vi "MFC Parse.vi"(1 "MFC Raw":fxp<+/-,24,9>[](array[numeric])=[0.0, 0.0, 0.0, 0.0, 0.0, 0.0, 0.0, 0.0, 0.0, 0.0, 0.0, 0.0, 0.0, 0.0, 0.0, 0.0, 0.0, 0.0, 0.0, 0.0, 0.0, 0.0, 0.0, 0.0, 0.0, 0.0, 0.0, 0.0, 0.0, 0.0, 0.0, 0.0, 0.0, 0.0, 0.0, 0.0, 0.0, 0.0, 0.0, 0.0, 0.0, 0.0, 0.0, 0.0, 0.0, 0.0, 0.0, 0.0, 0.0, 0.0, 0.0, 0.0, 0.0, 0.0, 0.0, 0.0, 0.0, 0.0, 0.0, 0.0, 0.0, 0.0, 0.0, 0.0, 0.0, 0.0, 0.0, 0.0, 0.0, 0.0, 0.0, 0.0, 0.0, 0.0, 0.0, 0.0, 0.0, 0.0, 0.0, 0.0, 0.0, 0.0, 0.0, 0.0, 0.0, 0.0, 0.0, 0.0, 0.0, 0.0, 0.0, 0.0, 0.0, 0.0, 0.0, 0.0, 0.0, 0.0, 0.0, 0.0, 0.0, 0.0, 0.0, 0.0, 0.0, 0.0, 0.0, 0.0, 0.0, 0.0, 0.0, 0.0, 0.0, 0.0, 0.0, 0.0, 0.0, 0.0, 0.0, 0.0, 0.0, 0.0, 0.0, 0.0, 0.0, 0.0, 0.0]) -> (0 "Array":dbl[](array[numeric]))   [LabVIEW 2014]
panel:
  out "MFC String 2":T1
  out "MFC Data 2":T2
  out "Array 2":dbl[](array[numeric])
  out "MFC Raw 2":fxp<+/-,24,9>[](array[numeric])
  out "AIR2":dbl
  out "AIR1":dbl
  out "MFC Data":T2
  out "AIR2  String":string
  out "AIR1 String":string
  out "MFC STRIING DATA":T1
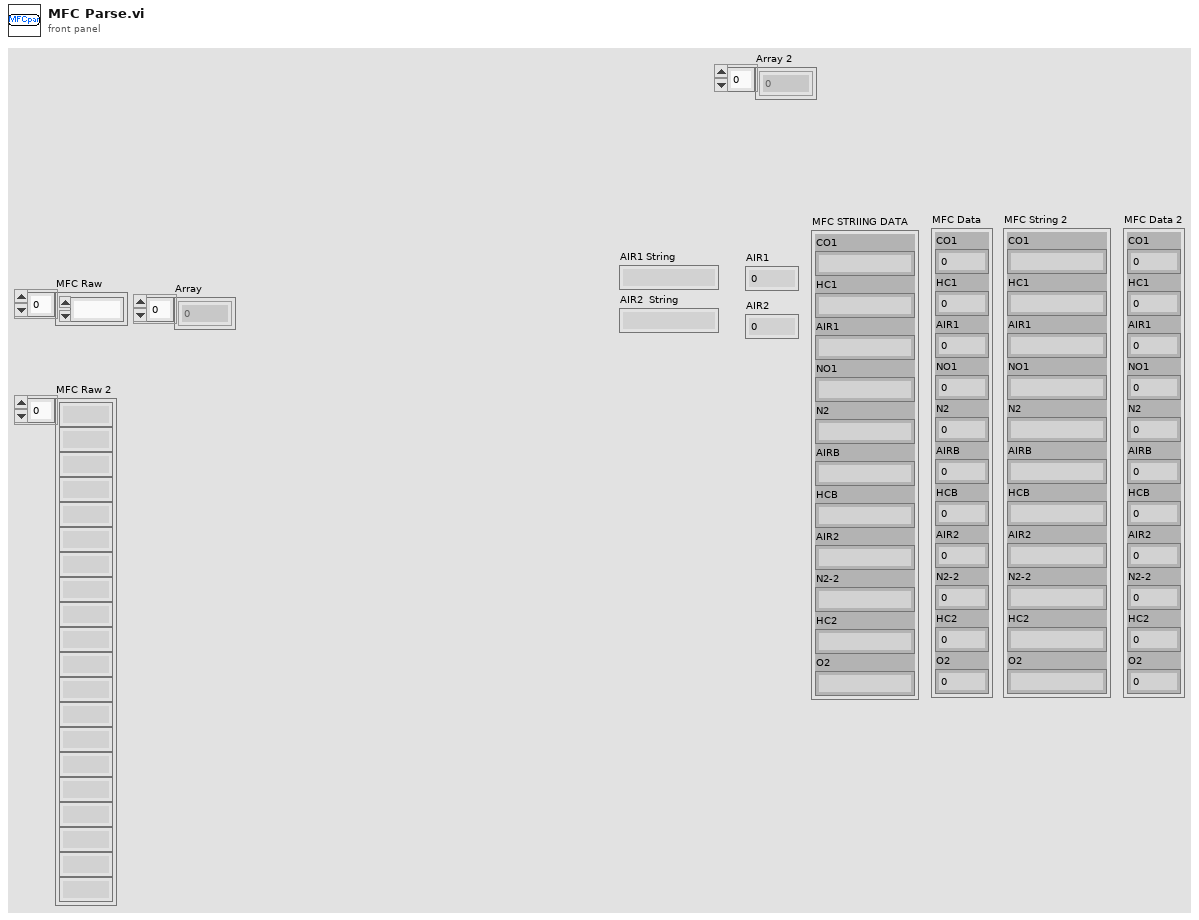
[diagram p1: front panel]
types:
  T1 = cluster{"CO1":string, "HC1":string, "AIR1":string, "NO1":string, "N2":string, "AIRB":string, "HCB":string, "AIR2":string, "N2-2":string, "HC2":string, "O2":string}
  T2 = cluster{"CO1":dbl, "HC1":dbl, "AIR1":dbl, "NO1":dbl, "N2":dbl, "AIRB":dbl, "HCB":dbl, "AIR2":dbl, "N2-2":dbl, "HC2":dbl, "O2":dbl}
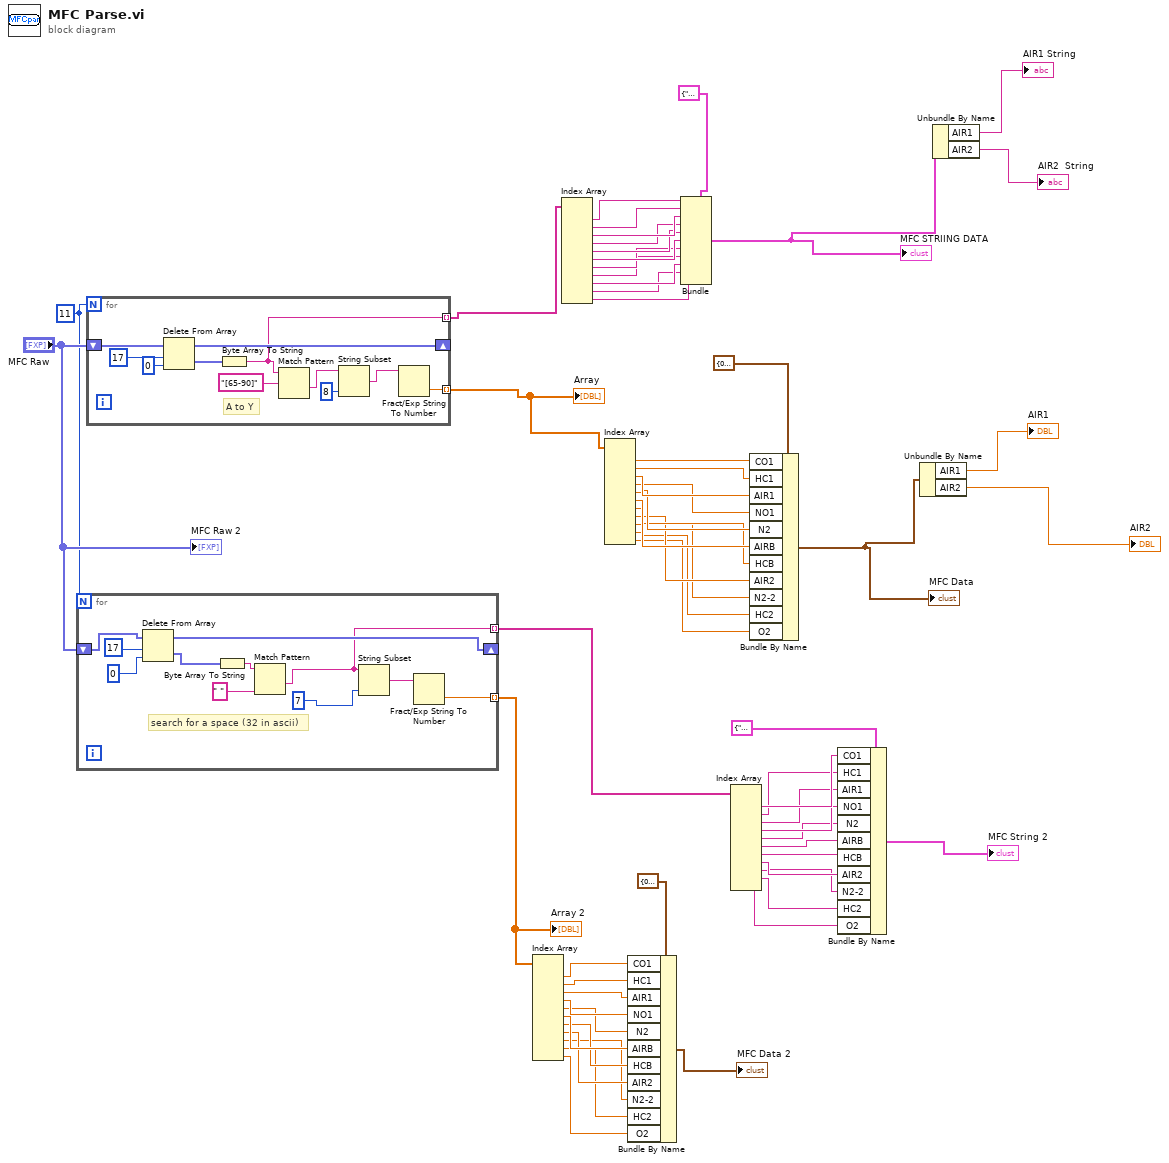
[diagram p0: block diagram]
diagram:
  w29 = 11
  n1 = for {
    N: w29 -> [_]
    shift-right: [w70] -> _
    shift-left: "MFC Raw" -> [w71]
    tunnel: [w64] -> w28 mode=indexing
    tunnel: [w63] -> w14 mode=indexing
    # "search for a space (32 in ascii)"
    n2 = Delete From Array(array=w71, length=17, index=0) -> (deleted portion=w69:fxp<+/-,24,9>[], array with subset deleted=w70:fxp<+/-,24,9>[])
    n3 = Byte Array To String(unsigned byte array=w69) -> (string=w68:string)
    n4 = Match Pattern(string=w68, regular expression=" ") -> (after substring=w63:string)  [unwired: 1 in, 3 out]
    n5 = String Subset(string=w63, length (rest)=7 ("offset (0)")) -> (substring=w65:string)  [unwired: 1 in]
    n6 = Fract/Exp String To Number(string=w65) -> (number=w64:dbl)  [unwired: 3 in, 1 out]
  }
  "Array 2" <- w28
  n7 = for {
    N: w29 -> [_]
    shift-right: [w76] -> _
    shift-left: "MFC Raw" -> [w84]
    tunnel: [w78] -> w46 mode=indexing
    tunnel: [w74] -> w62 mode=indexing
    # "A to Y"
    n8 = Delete From Array(array=w84, length=17, index=0) -> (deleted portion=w77:fxp<+/-,24,9>[], array with subset deleted=w76:fxp<+/-,24,9>[])
    n9 = Byte Array To String(unsigned byte array=w77) -> (string=w74:string)
    n10 = Match Pattern(string=w74, regular expression="[65-90]" ("search string")) -> (after substring=w81:string)  [unwired: 1 in, 3 out]
    n11 = String Subset(string=w81, length (rest)=8 ("length (rest)")) -> (substring=w79:string)  [unwired: 1 in]
    n12 = Fract/Exp String To Number(string=w79) -> (number=w78:dbl)  [unwired: 3 in, 1 out]
  }
  "Array" <- w46
  n13 = Index Array(array=w28) -> (element #1=w26:dbl, element #2=w25:dbl, element #3=w24:dbl, element #4=w23:dbl, element #5=w22:dbl, element #6=w21:dbl, element #7=w20:dbl, element #8=w19:dbl, element #9=w18:dbl, element #10=w17:dbl, element #11=w16:dbl)  [unwired: 11 in]
  n14 = Index Array(array=w62) -> (element #1=w60:string, element #2=w59:string, element #3=w58:string, element #4=w57:string, element #5=w56:string, element #6=w55:string, element #7=w54:string, element #8=w53:string, element #9=w52:string, element #10=w51:string, element #11=w50:string)  [unwired: 11 in]
  n15 = Index Array(array=w46) -> (element #1=w44:dbl, element #2=w43:dbl, element #3=w42:dbl, element #4=w41:dbl, element #5=w40:dbl, element #6=w39:dbl, element #7=w38:dbl, element #8=w37:dbl, element #9=w36:dbl, element #10=w35:dbl, element #11=w34:dbl)  [unwired: 11 in]
  n16 = Bundle By Name(cluster=T2 {"CO1"=0.0, "HC1"=0.0, "AIR1"=0.0, "NO1"=0.0, "N2"=0.0, "AIRB"=0.0, "HCB"=0.0, "AIR2"=0.0, "N2-2"=0.0, "HC2"=0.0, "O2"=0.0}, "CO1"=w26, "HC1"=w25, "AIR1"=w24, "NO1"=w23, "N2"=w22, "AIRB"=w21, "HCB"=w20, "AIR2"=w19, "N2-2"=w18, "HC2"=w17, "O2"=w16) -> (→"MFC Data 2":T2)
  n17 = Bundle(cluster=T1 {"CO1"="", "HC1"="", "AIR1"="", "NO1"="", "N2"="", "AIRB"="", "HCB"="", "AIR2"="", "N2-2"="", "HC2"="", "O2"=""}, "CO1"=w60, "HC1"=w59, "AIR1"=w58, "NO1"=w57, "N2"=w56, "AIRB"=w55, "HCB"=w54, "AIR2"=w53, "N2-2"=w52, "HC2"=w51, "O2"=w50) -> (w49:T1)
  "MFC STRIING DATA" <- w49
  n18 = Index Array(array=w14) -> (element #1=w12:string, element #2=w11:string, element #3=w10:string, element #4=w9:string, element #5=w8:string, element #6=w7:string, element #7=w6:string, element #8=w5:string, element #9=w4:string, element #10=w3:string, element #11=w2:string)  [unwired: 11 in]
  n19 = Bundle By Name(cluster=T2 {"CO1"=0.0, "HC1"=0.0, "AIR1"=0.0, "NO1"=0.0, "N2"=0.0, "AIRB"=0.0, "HCB"=0.0, "AIR2"=0.0, "N2-2"=0.0, "HC2"=0.0, "O2"=0.0}, "CO1"=w44, "HC1"=w43, "AIR1"=w42, "NO1"=w41, "N2"=w40, "AIRB"=w39, "HCB"=w38, "AIR2"=w37, "N2-2"=w36, "HC2"=w35, "O2"=w34) -> (w33:T2)
  "MFC Data" <- w33
  n20 = Bundle By Name(cluster=T1 {"CO1"="", "HC1"="", "AIR1"="", "NO1"="", "N2"="", "AIRB"="", "HCB"="", "AIR2"="", "N2-2"="", "HC2"="", "O2"=""}, "CO1"=w12, "HC1"=w11, "AIR1"=w10, "NO1"=w9, "N2"=w8, "AIRB"=w7, "HCB"=w6, "AIR2"=w5, "N2-2"=w4, "HC2"=w3, "O2"=w2) -> (→"MFC String 2":T1)
  n21 = Unbundle By Name(w33) -> ("AIR1"=→"AIR1":dbl, "AIR2"=→"AIR2":dbl)
  n22 = Unbundle By Name(w49) -> ("AIR1"=→"AIR1 String":string, "AIR2"=→"AIR2  String":string)
  "MFC Raw 2" <- "MFC Raw"
